vi "Enqueue Request Message.vi"(8 "error in (no error)":errorcluster, 9 "Message Data":variant, 10 "Message":string, 11 "Process In":refnum<class "Debug View.lvclass">) -> (0 "error out":errorcluster, 3 "Process Out":refnum<class "Debug View.lvclass">)   [LabVIEW 2020]
uses:
  Debug View.lvclass
  Debug View.lvclass/Debug View.ctl
  Protected/Messaging/Request Message Cluster.ctl
  Protected/Messaging/Message Cluster.ctl
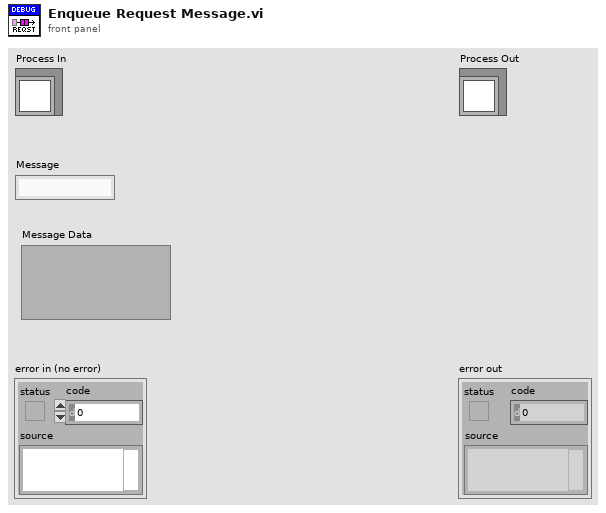
[diagram p1: front panel]
types:
  T1 = typedef "Debug View.lvclass/Request Message Cluster.ctl" = cluster{"Message":string, "Message Data":variant, "Request Error":errorcluster}
  T2 = typedef "Debug View.lvclass/Message Cluster.ctl" = cluster{"Message":string, "Message Data":variant, "Request Notifier":refnum<notifier>}
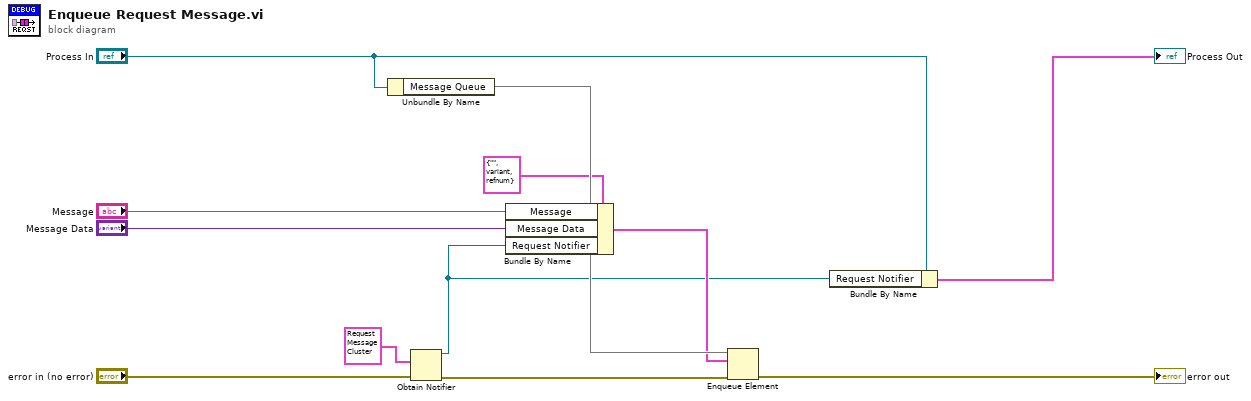
[diagram p0: block diagram]
diagram:
  n1 = Unbundle By Name("Process In") -> ("Message Queue"=w6)
  n2 = Obtain Notifier(notification data type=T1 {"Message"="", "Message Data"=variant, "Request Error"={"status"=FALSE, "code"=0, "source"=""}} ("Message Cluster"), error in (no error)="error in (no error)") -> (notifier out=w2:refnum<notifier>, error out=w1:errorcluster)  [unwired: 2 in, 1 out]
  n3 = Bundle By Name(cluster=T2 {"Message"="", "Message Data"=variant, "Request Notifier"=refnum} ("Message Cluster"), "Message"="Message", "Message Data"="Message Data", "Request Notifier"=w2) -> (w5:T2)
  n4 = Enqueue Element(queue=w6, element=w5, error in (no error)=w1) -> (error out=→"error out":errorcluster)  [unwired: 1 in, 2 out]
  n5 = Bundle By Name(cluster="Process In", "Request Notifier"=w2) -> (→"Process Out":cluster{})
